vi "Send Message to Owner.vi"(7 "GUID":string, 8 "error in (no error)":errorcluster, 9 "Message Payload":variant, 10 "Message":string, 11 "Attribute.Owner in":refnum<class "Attribute.Owner.lvclass">) -> (0 "error out":errorcluster, 3 "Attribute.Owner out":refnum<class "Attribute.Owner.lvclass">)   [LabVIEW 2021, in "smo.lvlib" / "Attribute.Owner.lvclass"]
uses:
  Attribute.Owner.lvclass
  Packet -- Cluster.ctl
  Attribute.Owner.lvclass/Attribute.Owner.ctl
  <vilib>/Utility/VariantDataType/VariantType.lvlib
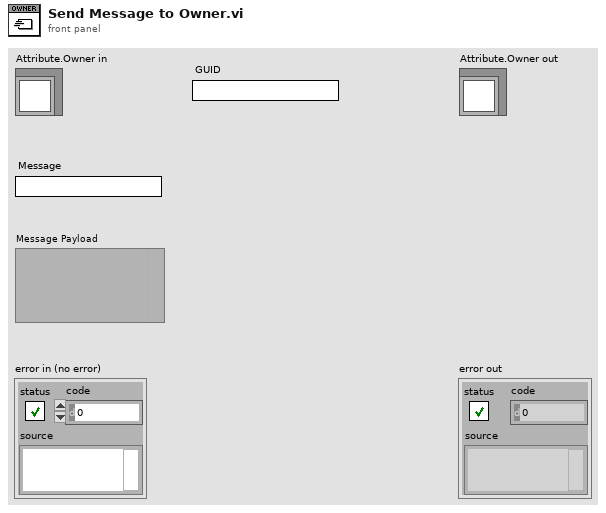
[diagram p1: front panel]
types:
  T1 = typedef "smo.lvlib/Attribute.Owner.lvclass/Packet -- Cluster.ctl" = cluster{"Message":string, "Payload":variant, "Source GUID":string}
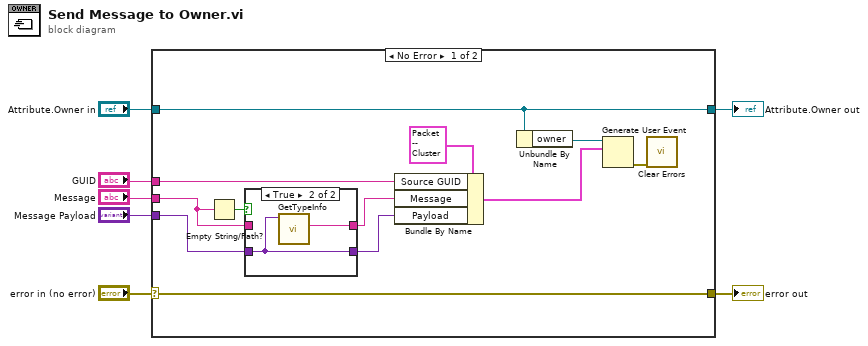
[diagram p0: block diagram]
diagram:
  n1 = case shown="No Error" "error in (no error)" {
    selector: "error in (no error)" -> [w19 w25]
    tunnel: [w19 w25] -> w6
    tunnel: [w16 w24] -> w4
    tunnel: "Attribute.Owner in" -> [w16 w24]
    tunnel: "Message Payload" -> [w11 _]
    tunnel: "Message" -> [w8 _]
    tunnel: "GUID" -> [w18 _]
    frame No Error {
      n2 = Empty String/Path?(string/path=w8) -> (empty?=w12:bool)
      n3 = case shown="True" w12 {
        tunnel: w11 -> [w20 w23]
        tunnel: [w20 w23] -> w10
        tunnel: [w21 w22] -> w9
        tunnel: w8 -> [w21 _]
        frame False {
        }
        frame True {
          n4 = call <vilib>:"GetTypeInfo.vi"("Variant"=w23) -> ("Name"=w22:string)  [unwired: 6 in, 4 out]
        }
      }
      n5 = Bundle By Name(cluster=T1 {"Message"="", "Payload"=variant, "Source GUID"=""} ("Packet"), "Source GUID"=w18, "Message"=w9, "Payload"=w10) -> (w14:T1)
      n6 = Unbundle By Name(w16) -> ("owner"=w15:refnum<user-event>)
      n7 = Generate User Event(user event=w15, event data cluster=w14) -> (error out=w13:errorcluster)  [unwired: 2 in, 1 out]
      n8 = call <vilib>:"Clear Errors.vi"("error in (no error)"=w13) -> ()  [unwired: 5 in, 2 out]
    }
    frame Error {
    }
  }
  "error out" <- w6
  "Attribute.Owner out" <- w4
